vi "AWS Worker.vi"(7 "System Message Queue In":refnum<queue>, 8 "error in (no error)":errorcluster) -> (0 "error out":errorcluster)   [LabVIEW 2019]
doc: "Uploads Summary or TDMS files (or both) in the specified file paths to an AWS S3 Bucket. This implementation uploads all files in the indicated path that match the designated file extention.\n\nNOTE: This VI renames the file to be uploaded to a temporary name to avoid potential conflicts with other processes writing to the same file. Since it uses the same temporary filename each time, this process is destructive to the local file(s). For Summary files, this is desirable, since the Summary file should always contain the most recent data. Future versions of this VI will include the option to archive the uploaded files locally, however that has not been implemented in this version. This version now includes error checking to handle instances where the AWS upload process reports an error. It will restore the filename of file that failed to upload and terminate the current upload session. The error is written to the system log and optionally, an email alert is issued. This version does not check validity of the uploaded file, it onlly responds to errors due to no internet connection, bad keys or bucket names, or error codes returned from AWS S3. \n\nCAUTION: Not recommended for uploading large (especially continuous) TDMS filess unless the network/internet connection has sufficient bandwidth, since the data may be generated faster than the transfer speed. Also, long file transfers might bog the system down and impact real time dertiminism of crtitical processes. \n\n\n2020 NREL"
uses:
  Globals and Definitions/System Message.ctl
  Globals and Definitions/Initialization Globals.vi
  Globals and Definitions/RT Globals RD v1.0.vi
  <vilib>/National Instruments/LabVIEW Interface for Amazon S3/LV Interface for Amazon S3.lvlib
panel:
  out "appended path":path
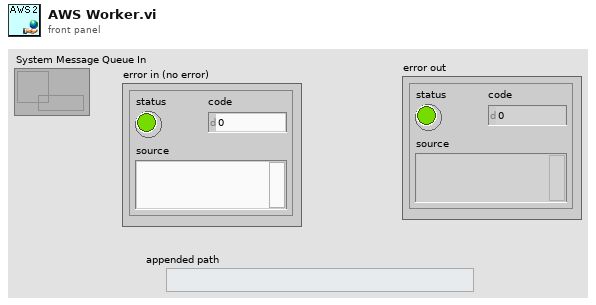
[diagram p1: front panel]
types:
  T1 = typedef "System Message.ctl" = cluster{"Message Tag":string, "Message Body":string, "Snooze Time (s)":dbl, "Snooze Alert?":bool, "Log Event?":bool, "Send Email":i32}
  T2 = cluster{"AWS Access Key":string, "AWS Secret Key":string}
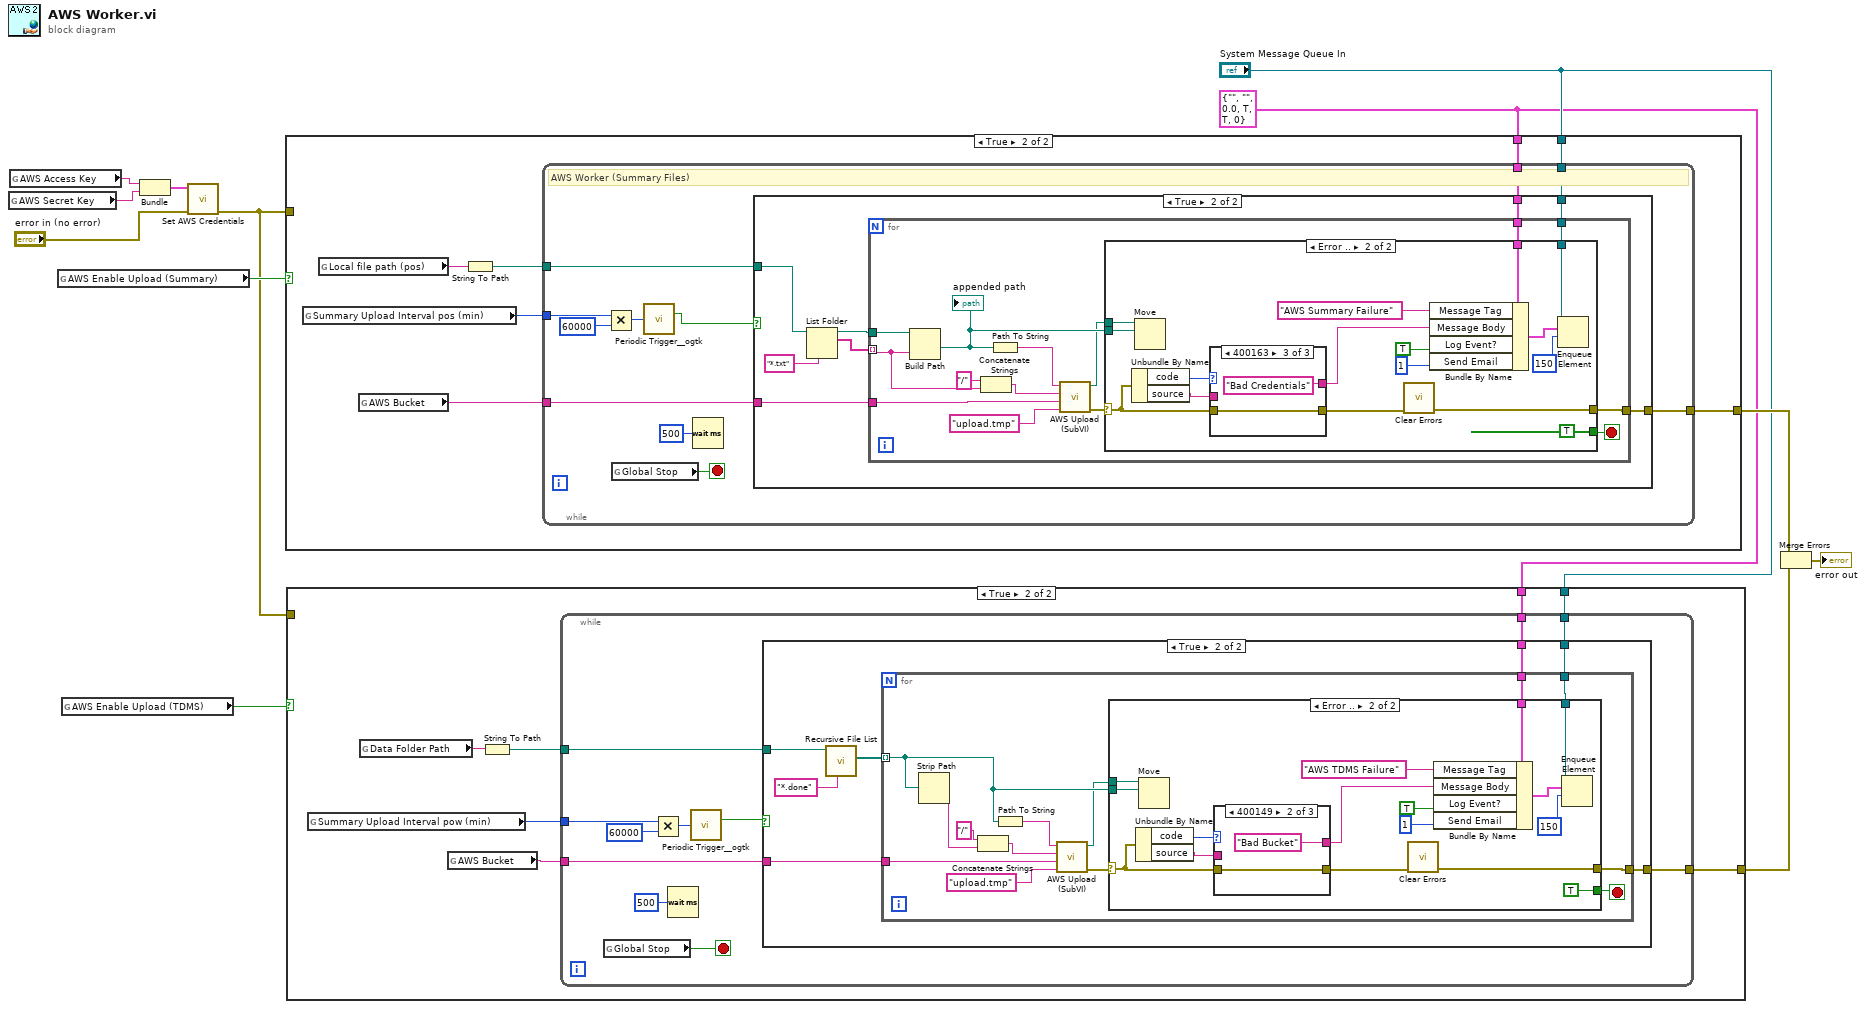
[diagram p0: block diagram]
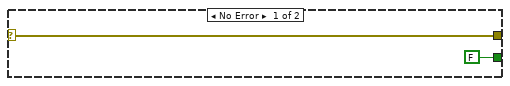
[diagram p4: hidden frame]
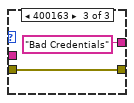
[diagram p6: hidden frame]
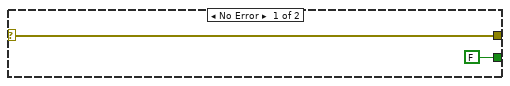
[diagram p9: hidden frame]
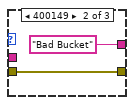
[diagram p11: hidden frame]
diagram:
  w2 = T1 {"Message Tag"="", "Message Body"="", "Snooze Time (s)"=0.0, "Snooze Alert?"=TRUE, "Log Event?"=TRUE, "Send Email"=0}
  n1 = global read "Initialization Globals.vi" "AWS Secret Key"() -> (w11:string)
  n2 = global read "Initialization Globals.vi" "AWS Access Key"() -> (w10:string)
  n3 = global read "Initialization Globals.vi" "AWS Enable Upload (Summary)"() -> (w9:bool)
  n4 = global read "Initialization Globals.vi" "AWS Enable Upload (TDMS)"() -> (w8:bool)
  n5 = Bundle("AWS Access Key"=w10, "AWS Secret Key"=w11) -> (w12:T2)  [unwired: 1 in]
  n6 = call <vilib>:"Set AWS Credentials.vi"("error in (no error)"="error in (no error)", "AWS Credentials in"=w12) -> ("error out"=w7:errorcluster)  [unwired: 9 in]
  n7 = case shown="True" w9 {
    tunnel: [w13 w18] -> w6
    tunnel: w7 -> [w13 _]
    tunnel: w2 -> [_ w15]
    tunnel: "System Message Queue In" -> [_ w14]
    frame False {
    }
    frame True {
      # "AWS Upload (Summary Files)"
      n8 = global read "Initialization Globals.vi" "Summary Upload Interval pos (min)"() -> (w20:i32)
      n9 = global read "Initialization Globals.vi" "Local file path (pos)"() -> (w17:string)
      n10 = global read "Initialization Globals.vi" "AWS Bucket"() -> (w19:string)
      n11 = String To Path(string=w17) -> (path=w16:path)
      n12 = while {
        tunnel: w20 -> [w26]
        tunnel: w19 -> [w25]
        tunnel: [w24] -> w18
        tunnel: w16 -> [w23]
        tunnel: w15 -> [w22]
        tunnel: w14 -> [w21]
        stop <- w27 stop-if-true
        # "AWS Worker (Summary Files)"
        n13 = Multiply(x=w26, y=60000) -> (x*y=w30:i32)
        n14 = global read "RT Globals RD v1.0.vi" "Global Stop"() -> (w27:bool)
        n15 = call <userlib>:"Periodic Trigger__ogtk.vi"("time (ms)"=w30) -> ("Triggered"=w28:bool)  [unwired: 12 in, 2 out]
        n16 = Wait (ms)(milliseconds to wait=u32 500) -> ()  [unwired: 1 out]
        n17 = case shown="True" w28 {
          tunnel: w25 -> [_ w39]
          tunnel: [_ w38] -> w24
          tunnel: w23 -> [_ w34]
          tunnel: w22 -> [_ w33]
          tunnel: w21 -> [_ w32]
          frame False {
          }
          frame True {
            n18 = List Folder(path=w34, pattern="*.txt") -> (path out=w35:path, filenames=w36:string[])  [unwired: 2 in, 2 out]
            n19 = for {
              tunnel: w36 -> [w49] mode=indexing
              tunnel: w35 -> [w53]
              tunnel: w39 -> [w50]
              tunnel: [w46] -> w38
              tunnel: w33 -> [w41]
              tunnel: w32 -> [w40]
              stop <- w42 stop-if-true
              n20 = Build Path(base path=w53, name or relative path=w49) -> (appended path=w45:path)
              "appended path" <- w45
              n21 = Concatenate Strings("/" ("string"), w49) -> (w47:string)
              n22 = Path To String(path=w45) -> (string=w51:string)
              n23 = call "AWS Upload (SubVI).vi"("Temp Filename"="upload.tmp", "AWS Bucket"=w50, "Object path"=w47, "Local File Path"=w51) -> ("error out"=w43:errorcluster, "Temp Path"=w44:path)  [unwired: 6 in]
              n24 = case shown="Error .." w43 {
                selector: w43 -> [w54 w64]
                tunnel: [w54 w71] -> w46
                tunnel: w45 -> [_ w67]
                tunnel: w44 -> [_ w66]
                tunnel: [FALSE TRUE] -> w42
                tunnel: w41 -> [_ w57]
                tunnel: w40 -> [_ w56]
                frame No Error {
                }
                frame Error {
                  n25 = Unbundle By Name(w64) -> ("code"=w69:i32, "source"=w68:string)
                  n26 = Move(source path=w66, 10:w67) -> ()  [unwired: 3 in, 3 out]
                  n27 = case shown="400163" w69 {
                    tunnel: [w73 w75 w77] -> w70
                    tunnel: w64 -> [w73 w75 w77]
                    tunnel: [w72 "Bad Bucket" "Bad Credentials"] -> w58
                    tunnel: w68 -> [w72 _ _]
                    frame 0, Default {
                    }
                    frame 400149 {
                    }
                    frame 400163 {
                    }
                  }
                  n28 = call <vilib>:"Clear Errors.vi"("error in (no error)"=w70) -> ("error out"=w71:errorcluster)  [unwired: 5 in, 1 out]
                  n29 = Bundle By Name(cluster=w57, "Message Tag"="AWS Summary Failure", "Message Body"=w58, "Log Event?"=TRUE, "Send Email"=1) -> (w60:T1)
                  n30 = Enqueue Element(queue=w56, element=w60, timeout in ms (-1)=150) -> ()  [unwired: 1 in, 3 out]
                }
              }
            }
          }
        }
      }
    }
  }
  n31 = case shown="True" w8 {
    tunnel: w7 -> [w78 _]
    tunnel: [w78 w83] -> w5
    tunnel: "System Message Queue In" -> [_ w80]
    tunnel: w2 -> [_ w79]
    frame False {
    }
    frame True {
      n32 = global read "Initialization Globals.vi" "Summary Upload Interval pow (min)"() -> (w84:i32)
      n33 = global read "Initialization Globals.vi" "Data Folder Path"() -> (w82:string)
      n34 = global read "Initialization Globals.vi" "AWS Bucket"() -> (w85:string)
      n35 = String To Path(string=w82) -> (path=w81:path)
      n36 = while {
        tunnel: w85 -> [w95]
        tunnel: w84 -> [w90]
        tunnel: [w89] -> w83
        tunnel: w81 -> [w88]
        tunnel: w80 -> [w87]
        tunnel: w79 -> [w86]
        stop <- w94 stop-if-true
        n37 = global read "RT Globals RD v1.0.vi" "Global Stop"() -> (w94:bool)
        n38 = Multiply(x=w90, y=60000) -> (x*y=w93:i32)
        n39 = Wait (ms)(milliseconds to wait=u32 500) -> ()  [unwired: 1 out]
        n40 = call <userlib>:"Periodic Trigger__ogtk.vi"("time (ms)"=w93) -> ("Triggered"=w91:bool)  [unwired: 12 in, 2 out]
        n41 = case shown="True" w91 {
          tunnel: w95 -> [_ w103]
          tunnel: [_ w102] -> w89
          tunnel: w88 -> [_ w100]
          tunnel: w87 -> [_ w98]
          tunnel: w86 -> [_ w97]
          frame False {
          }
          frame True {
            n42 = call <vilib>:"Recursive File List.vi"("pattern"="*.done", "Folder Path"=w100) -> ("All Files in Dir"=w99:path[])  [unwired: 5 in, 4 out]
            n43 = for {
              tunnel: w103 -> [w114]
              tunnel: [w109] -> w102
              tunnel: w99 -> [w108] mode=indexing
              tunnel: w98 -> [w106]
              tunnel: w97 -> [w105]
              stop <- w104 stop-if-true
              n44 = Strip Path(path=w108) -> (name=w111:string)  [unwired: 1 out]
              n45 = Concatenate Strings("/" ("string"), w111) -> (w112:string)
              n46 = Path To String(path=w108) -> (string=w115:string)
              n47 = call "AWS Upload (SubVI).vi"("Temp Filename"="upload.tmp", "AWS Bucket"=w114, "Object path"=w112, "Local File Path"=w115) -> ("error out"=w110:errorcluster, "Temp Path"=w107:path)  [unwired: 6 in]
              n48 = case shown="Error .." w110 {
                selector: w110 -> [w117 w127]
                tunnel: [w117 w134] -> w109
                tunnel: w108 -> [_ w130]
                tunnel: w107 -> [_ w129]
                tunnel: [FALSE TRUE] -> w104
                tunnel: w105 -> [_ w120]
                tunnel: w106 -> [_ w119]
                frame No Error {
                }
                frame Error {
                  n49 = Unbundle By Name(w127) -> ("code"=w132:i32, "source"=w131:string)
                  n50 = Move(source path=w129, 10:w130) -> ()  [unwired: 3 in, 3 out]
                  n51 = case shown="400149" w132 {
                    tunnel: [w136 w138 w140] -> w133
                    tunnel: w127 -> [w136 w138 w140]
                    tunnel: [w135 "Bad Bucket" "Bad Credentials"] -> w121
                    tunnel: w131 -> [w135 _ _]
                    frame 0, Default {
                    }
                    frame 400149 {
                    }
                    frame 400163 {
                    }
                  }
                  n52 = call <vilib>:"Clear Errors.vi"("error in (no error)"=w133) -> ("error out"=w134:errorcluster)  [unwired: 5 in, 1 out]
                  n53 = Bundle By Name(cluster=w120, "Message Tag"="AWS TDMS Failure", "Message Body"=w121, "Log Event?"=TRUE, "Send Email"=1) -> (w123:T1)
                  n54 = Enqueue Element(queue=w119, element=w123, timeout in ms (-1)=150) -> ()  [unwired: 1 in, 3 out]
                }
              }
            }
          }
        }
      }
    }
  }
  n55 = Merge Errors(w6, w5) -> (→"error out":errorcluster)
